vi "WritePanelData_test_ringsgreyedcorrect.vi"(8 "error in (no error)":errorcluster, 11 "Maui.Test.DefaultDirectory in":refnum<class "Maui.Test.DefaultDirectory.lvclass">) -> (0 "error out":errorcluster, 3 "Maui.Test.DefaultDirectory out":refnum<class "Maui.Test.DefaultDirectory.lvclass">)   [LabVIEW 2020, in "Maui.Test.DefaultDirectory.lvclass"]
uses:
  Maui.Test.DefaultDirectory.lvclass
  Maui.Test.DefaultDirectory.lvclass/Maui.Test.DefaultDirectory.ctl
  <vilib>/addons/_JKI Toolkits/Caraya/classes/Assert/Assert Equal Value_Variant.vi
  <vilib>/addons/_JKI Toolkits/Caraya/classes/Test/Test.lvclass
  <vilib>/addons/_JKI Toolkits/Caraya/classes/Assert/Assert.lvclass
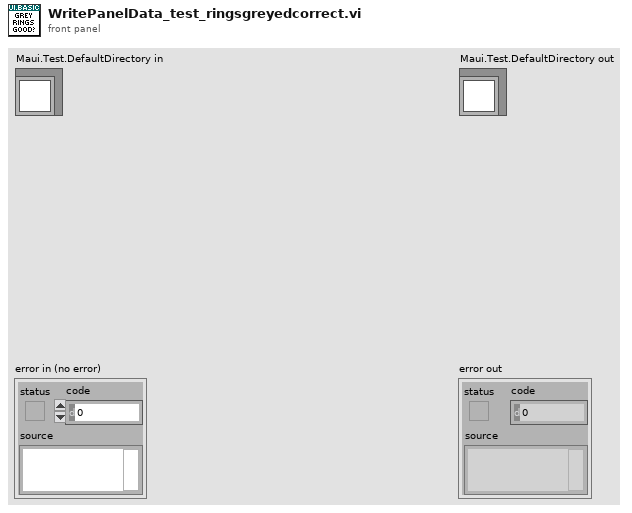
[diagram p1: front panel]
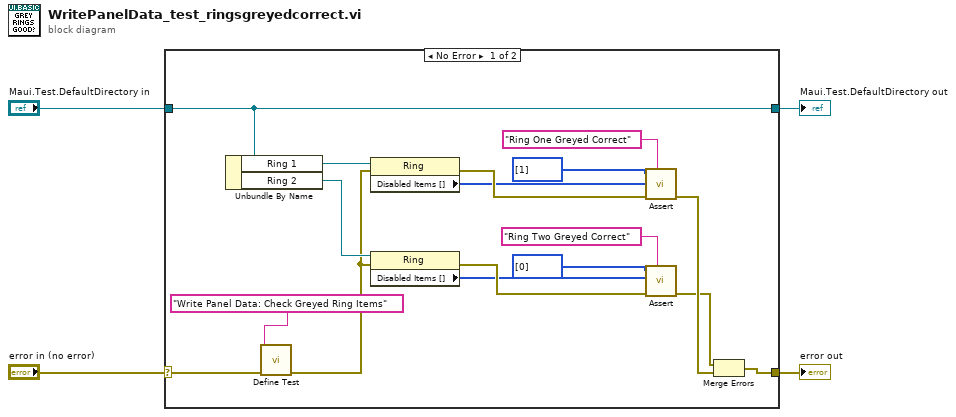
[diagram p0: block diagram]
diagram:
  n1 = case shown="No Error" "error in (no error)" {
    selector: "error in (no error)" -> [w18 w23]
    tunnel: [w17 w23] -> w3
    tunnel: [w21 w22] -> w1
    tunnel: "Maui.Test.DefaultDirectory in" -> [w21 w22]
    frame No Error {
      n2 = Unbundle By Name(w21) -> ("Ring 1"=w15:refnum<vi>, "Ring 2"=w6:refnum<vi>)
      n3 = call <vilib>:"Define Test.vi"("error in (no error)"=w18, "Label (VI Title)"="Write Panel Data: Check Greyed Ring Items") -> ("error out"=w5:errorcluster)  [unwired: 9 in]
      n4 = property class="Ring"(reference=w15, error in=w5) -> (error out=w14:errorcluster, "Disabled Items []"=w13:i32[])  [unwired: 1 out]
      n5 = property class="Ring"(reference=w6, error in=w5) -> (error out=w8:errorcluster, "Disabled Items []"=w7:i32[])  [unwired: 1 out]
      n6 = call-poly <vilib>:"Assert.vi"("Label"="Ring One Greyed Correct" ("Label (VI Title)"), "error in (no error)"=w14, "Y"=w13, "X"=i32[] [1]) -> ("error out"=w19:errorcluster)  [unwired: 7 in]
      n7 = call-poly <vilib>:"Assert.vi"("Label"="Ring Two Greyed Correct" ("Label (VI Title)"), "error in (no error)"=w8, "Y"=w7, "X"=i32[] [0]) -> ("error out"=w9:errorcluster)  [unwired: 7 in]
      n8 = Merge Errors(w9, w19) -> (w17:errorcluster)
    }
    frame Error {
    }
  }
  "error out" <- w3
  "Maui.Test.DefaultDirectory out" <- w1
